vi "Stop Core.vi"(10 "final error code":i32, 11 "IMAQdx Actor in":refnum<class "IMAQdx Actor.lvclass">) -> (3 "IMAQdx Actor out":refnum<class "IMAQdx Actor.lvclass">)   [LabVIEW 2014, in "IMAQdx Actor.lvlib" / "IMAQdx Actor.lvclass"]
doc: "(<B>Filename</B>: Actor Framework.lvlib:Actor.lvclass:Stop Core.vi)\n\nDefines what the actor does before it stops. Use the <B>final error code</B> input to determine whether the actor shut down in response to an error.\n\nBy default, this method does nothing. A descendant class may override it to define behavior, such as shutting down any processes the actor initiated in its override of the Actor Core method."
uses:
  IMAQdx Actor.lvclass
  Operation Mode.ctl
  IMAQdx Actor.lvclass/IMAQdx Actor.ctl
  Camera Actor/Camera Actor/Camera Actor.lvclass
  IMAQdx Actor.lvlib
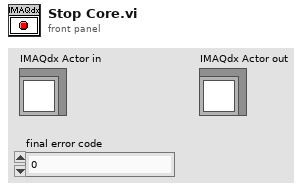
[diagram p1: front panel]
types:
  T1 = typedef "IMAQdx Actor.lvlib/Operation Mode.ctl" = enum16{"Acquisition", "Break", "Exit"}
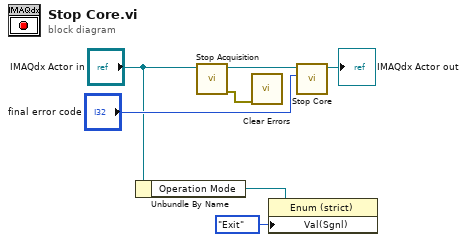
[diagram p0: block diagram]
diagram:
  n1 = Unbundle By Name("IMAQdx Actor in") -> ("Operation Mode"=w5:refnum<vi>)
  n2 = call-dynamic "Stop Acquisition.vi"("IMAQdx Actor in"="IMAQdx Actor in") -> ("error out"=w1:errorcluster, "IMAQdx Actor out"=w2:refnum<class "IMAQdx Actor.lvclass">)  [unwired: 9 in]
  n3 = call <vilib>:"Clear Errors.vi"("error in (no error)"=w1) -> ()  [unwired: 5 in, 2 out]
  n4 = property class="Enum (strict)"(reference=w5, "Val(Sgnl)"=Operation_Mode."Exit" ("Value (Signaling)")) -> ()  [unwired: 1 in, 2 out]
  n5 = call-parent "Stop Core.vi"("final error code"="final error code", "Actor in"=w2) -> ("Actor out"=→"IMAQdx Actor out":refnum<class "IMAQdx Actor.lvclass">)  [unwired: 9 in]
